vi "ReadUDP.vi"() -> ()   [LabVIEW 2012]
panel:
  out "Current Position":dbl[](array[numeric])
  in  "stop":bool
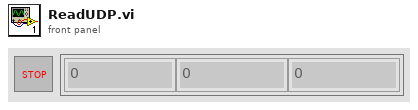
[diagram p1: front panel]
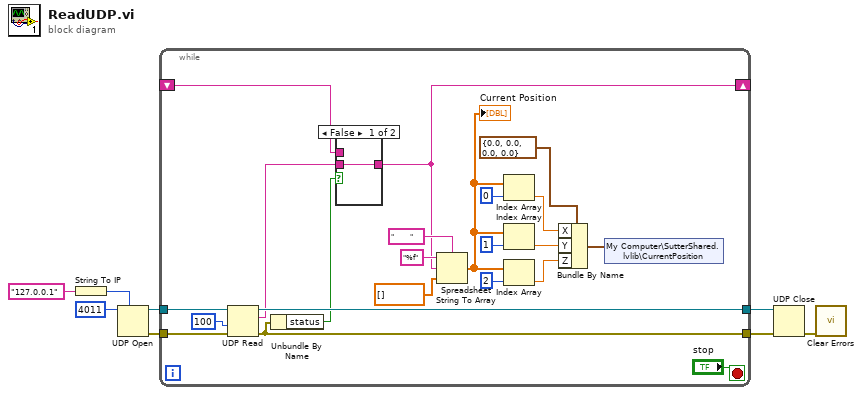
[diagram p0: block diagram]
diagram:
  n1 = String To IP(1:"127.0.0.1" ("name")) -> (0:w6:u32)
  n2 = UDP Open(7:w6, 11:u16 4011 ("port")) -> (port=w2:refnum<k16>, 0:w7:errorcluster)  [unwired: 3 in, 1 out]
  n3 = while {
    tunnel: w2 -> [w30]
    tunnel: [w29] -> w3
    shift-right: [w9] -> _
    shift-left: _ -> [w26]
    tunnel: w7 -> [w25]
    tunnel: [w24] -> w8
    stop <- "stop" stop-if-true
    n4 = UDP Read(connection ID=w30, timeout ms (25000)=100, 8:w25) -> (data out=w27:string, error out=w24:errorcluster, 3:w29:refnum<k16>)  [unwired: 1 in, 2 out]
    n5 = Unbundle By Name(w24) -> ("status"=w28:bool)
    n6 = case shown="False" w28 {
      tunnel: w27 -> [w31 _]
      tunnel: [w31 w32] -> w9
      tunnel: w26 -> [_ w32]
      frame False {
      }
      frame True {
      }
    }
    n7 = Spreadsheet String To Array(delimiter (Tab)="        ", format string="%f", spreadsheet string=w9, array type (2D Dbl)=dbl[] []) -> (array=w10:dbl[])
    "Current Position" <- w10
    n8 = Index Array(array=w10, index=0) -> (element=w19:dbl)
    n9 = Index Array(array=w10, index=1) -> (element=w18:dbl)
    n10 = Index Array(array=w10, index=2) -> (element=w17:dbl)
    n11 = Bundle By Name(cluster=cluster{"X":dbl, "Y":dbl, "Z":dbl, "Depth":dbl} {"X"=0.0, "Y"=0.0, "Z"=0.0, "Depth"=0.0}, "X"=w19, "Y"=w18, "Z"=w17) -> (w21:cluster{"X":dbl, "Y":dbl, "Z":dbl, "Depth":dbl})
    n12 = shared-variable "My Computer\\SutterShared.lvlib\\CurrentPosition"(w21) -> ()  [unwired: 1 in, 1 out]
  }
  n13 = UDP Close(connection ID=w3, 8:w8) -> (error out=w1:errorcluster)  [unwired: 1 out]
  n14 = call <vilib>:"Clear Errors.vi"("error in (no error)"=w1) -> ()  [unwired: 6 in, 1 out]
